vi "rx_init.vi"(8 "error in (no error)":errorcluster, 9 "Queues in":T1, 10 "Modulation Parameters In":T3 {"RX Parameters"."RX Sample Rate" items=["4M"]}, 11 "HW parameters In":T2={"Device IP Address"="192.168.11.6", "Active Antenna"="RX1", "Carrier Frequency (Hz)"=915000000.0, "Gain (dB)"=10.0, "Trigger Level"=0.01, "Bandwidth (Hz)"=40000000.0, "Reference Position (%)"=10.0, "Capture Time (s)"=0.0004, "Simulate"=FALSE} {"Capture Time (s)" format="%.2p"; "Bandwidth (Hz)" format="%.2p"; "Trigger Level" format="%#.3p"; "Gain (dB)" format="%.2f"; "Carrier Frequency (Hz)" format="%.2p"}) -> (0 "error out":errorcluster, 1 "Queues out":T1, 2 "Modulation Parameters Out":T3 {"RX Parameters"."RX Sample Rate" items=["4M"]}, 3 "HW parameters Out":T2={"Device IP Address"="192.168.11.6", "Active Antenna"="RX1", "Carrier Frequency (Hz)"=915000000.0, "Gain (dB)"=10.0, "Trigger Level"=0.01, "Bandwidth (Hz)"=40000000.0, "Reference Position (%)"=10.0, "Capture Time (s)"=0.0004, "Simulate"=FALSE} {"Capture Time (s)" format="%.2p"; "Bandwidth (Hz)" format="%.2p"; "Trigger Level" format="%#.3p"; "Gain (dB)" format="%.2f"; "Carrier Frequency (Hz)" format="%.2p"})   [LabVIEW 2012, in "gds_hw_config.lvlib"]
uses:
  EE 497/LABS/SDR/control_type_defs.llb/rx_hw params.ctl
  EE 497/LABS/SDR/control_type_defs.llb/Queues.ctl
  gds_hw_config.lvlib
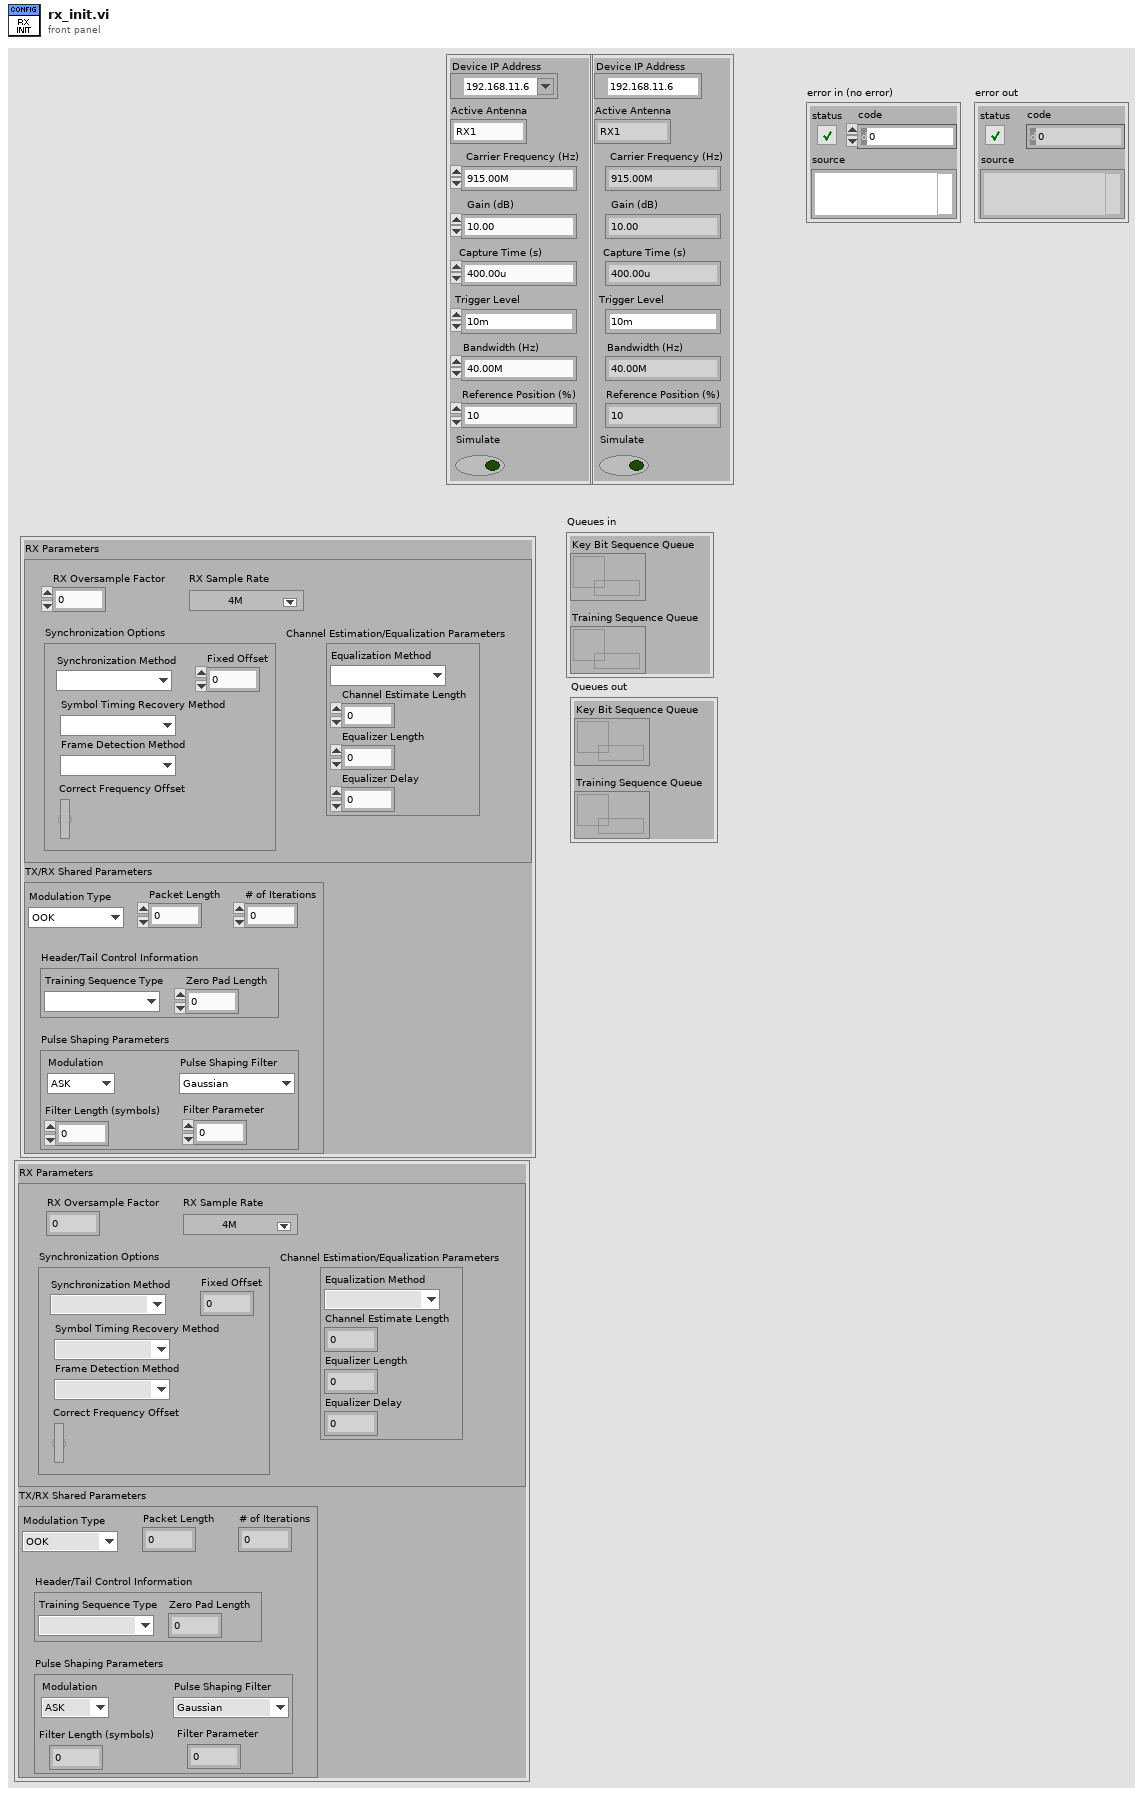
[diagram p1: front panel]
types:
  T1 = typedef "Queues.ctl" = cluster{"Key Bit Sequence Queue":refnum<queue>, "Training Sequence Queue":refnum<queue>}
  T2 = typedef "rx_hw params.ctl" = cluster{"Device IP Address":refnum<k15>, "Active Antenna":string, "Carrier Frequency (Hz)":dbl, "Gain (dB)":dbl, "Trigger Level":dbl, "Bandwidth (Hz)":dbl, "Reference Position (%)":dbl, "Capture Time (s)":dbl, "Simulate":bool}
  T3 = cluster{"RX Parameters":cluster{"RX Oversample Factor":dbl, "RX Sample Rate":u16, "Synchronization Options":cluster{"Synchronization Method":enum16{""}, "Symbol Timing Recovery Method ":enum16{""}, "Fixed Offset":dbl, "Frame Detection Method":enum16{""}, "Correct Frequency Offset":bool}, "Channel Estimation/Equalization Parameters":cluster{"Equalization Method":enum16{""}, "Channel Estimate Length":dbl, "Equalizer Length":dbl, "Equalizer Delay":dbl}}, "TX/RX Shared Parameters":cluster{"Modulation Type":enum16{"OOK", "FSK"}, "Packet Length":dbl, "# of Iterations":dbl, "Pulse Shaping Parameters":cluster{"Modulation":enum16{"ASK", "FSK", "PSK", "QAM", "MSK", "PAM"}, "Pulse Shaping Filter":enum16{"Gaussian"}, "Filter Length (symbols)":dbl, "Filter Parameter":dbl}, "Header/Tail Control Information":cluster{"Training Sequence Type":enum16{""}, "Zero Pad Length":dbl}}}
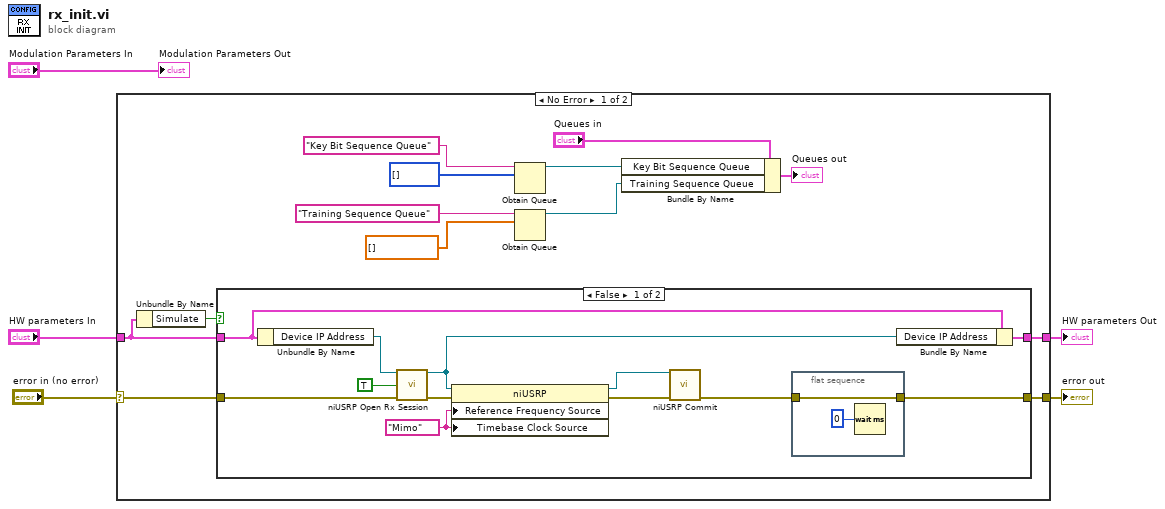
[diagram p0: block diagram]
diagram:
  n1 = case shown="No Error" "error in (no error)" {
    selector: "error in (no error)" -> [w17 w35]
    tunnel: "HW parameters In" -> [w16 w36]
    tunnel: [w15 w36] -> w2
    tunnel: [w14 w35] -> w1
    frame No Error {
      n2 = Unbundle By Name(w16) -> ("Simulate"=w18:bool)
      n3 = case shown="False" w18 {
        tunnel: w17 -> [w27 w33]
        tunnel: w16 -> [w28 w34]
        tunnel: [w26 w34] -> w15
        tunnel: [w19 w33] -> w14
        frame False {
          w23 = "Mimo" ("Clocking and Synchronization:Reference Frequency Source")
          n4 = Unbundle By Name(w28) -> ("Device IP Address"=w30:refnum<k15>)
          n5 = call <instrlib>:"niUSRP Open Rx Session.vi"("device names"=w30, "reset"=TRUE, "error in (no error)"=w27) -> ("session handle out"=w24:refnum<k15>, "error out"=w25:errorcluster)  [unwired: 11 in]
          n6 = property class="niUSRP"(reference=w24, error in=w25, "Reference Frequency Source"=w23, "Timebase Clock Source"=w23) -> (reference out=w22:refnum<k15>, error out=w21:errorcluster)
          n7 = call <instrlib>:"niUSRP Commit.vi"("session handle"=w22, "error in (no error)"=w21) -> ("error out"=w20:errorcluster)  [unwired: 12 in, 1 out]
          n8 = flat-sequence {
            tunnel: [w31] -> w19
            tunnel: w20 -> [w31]
            frame #0 {
              n9 = Wait (ms)(milliseconds to wait=u32 0) -> ()  [unwired: 1 out]
            }
          }
          n10 = Bundle By Name(cluster=w28, "Device IP Address"=w24) -> (w26:T2)
        }
        frame True {
        }
      }
      n11 = Obtain Queue(name (unnamed)="Key Bit Sequence Queue", element data type=u8[] []) -> (queue out=w9:refnum<queue>)  [unwired: 3 in, 2 out]
      n12 = Obtain Queue(name (unnamed)="Training Sequence Queue", element data type=cdb[] []) -> (queue out=w8:refnum<queue>)  [unwired: 3 in, 2 out]
      n13 = Bundle By Name(cluster="Queues in", "Key Bit Sequence Queue"=w9, "Training Sequence Queue"=w8) -> (→"Queues out":T1)
    }
    frame Error {
    }
  }
  "error out" <- w1
  "HW parameters Out" <- w2
  "Modulation Parameters Out" <- "Modulation Parameters In"
